vi "Rearrange image (20-02-2018).vi"(7 "Reference position":T2, 8 "error in (no error)":errorcluster, 9 "String ref array":refnum<vi>[](array[refnum]), 10 "Image refnum array":refnum<vi>[](array[refnum]), 11 "Image resize cluster":T3={"Image array"=[{"Size"={"Width"=500, "Height"=400}, "Position"={"Left"=0, "Top"=0}}, {"Size"={"Width"=500, "Height"=400}, "Position"={"Left"=0, "Top"=440}}, {"Size"={"Width"=500, "Height"=840}, "Position"={"Left"=505, "Top"=0}}], "String array"=[{"Size"={"Width"=503, "Height"=30}, "Position"={"Left"=0, "Top"=-30}}, {"Size"={"Width"=503, "Height"=30}, "Position"={"Left"=0, "Top"=410}}, {"Size"={"Width"=503, "Height"=30}, "Position"={"Left"=505, "Top"=-30}}]}) -> (0 "error out (no error)":errorcluster)   [LabVIEW 2015]
uses:
  Type Definitions/Controls and Indicators/String2.ctl
  <vilib>/Utility/miscctls.llb/LVPositionTypeDef.ctl
  <vilib>/Utility/miscctls.llb/LVBoundsTypeDef.ctl
  ZenGage v3.0 UI.lvclass
panel:
  out "Top Left 5":T4(plugin-control)
  out "Top Left 6":T5
  out "Top Left 3":T4(plugin-control)
  out "Top Left 4":T5
  out "Top Left 2":T4(plugin-control)
  out "Top Left":T5
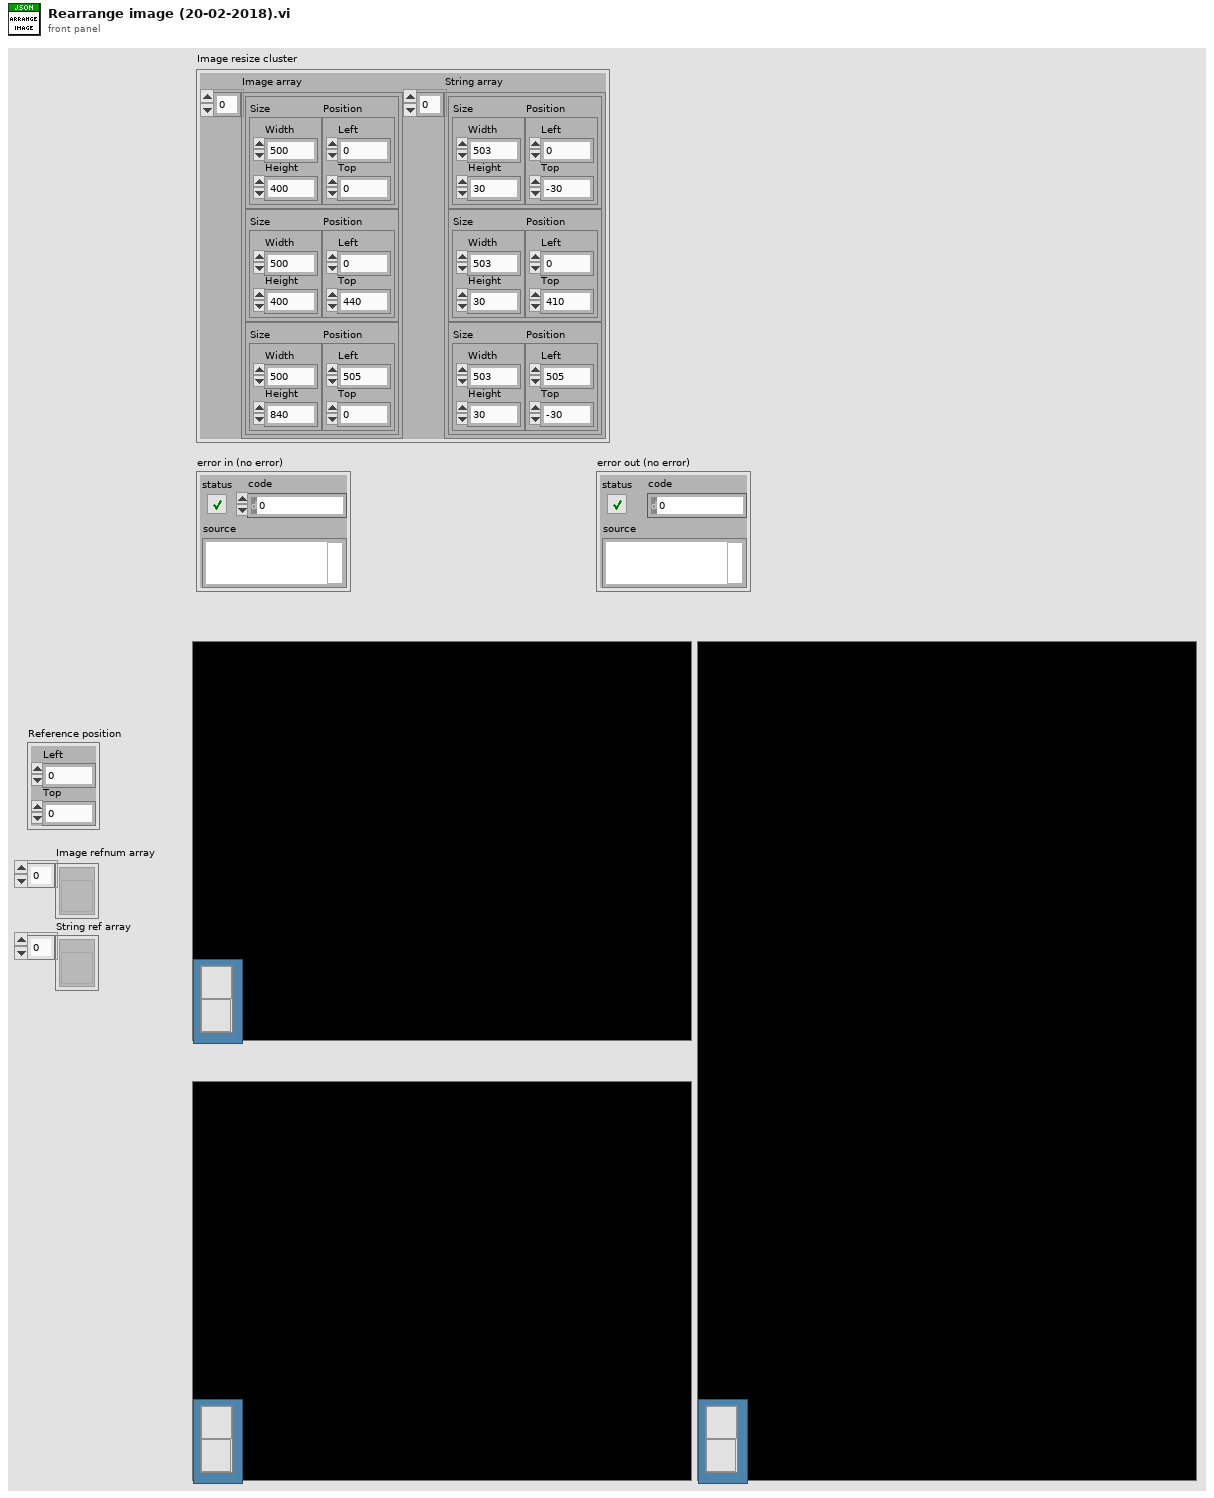
[diagram p1: front panel]
types:
  T1 = typedef "LVBoundsTypeDef.ctl" = cluster{"Width":u32, "Height":u32}
  T2 = typedef "LVPositionTypeDef.ctl" = cluster{"Left":i32, "Top":i32}
  T3 = cluster{"Image array":cluster{"Size":T1, "Position":T2}[], "String array":cluster{"Size":T1, "Position":T2}[]}
  T4 = typedef "IMAQ Image.ctl" = refnum<image>
  T5 = typedef "ZenGage v3.0 UI.lvclass/String2.ctl" = string
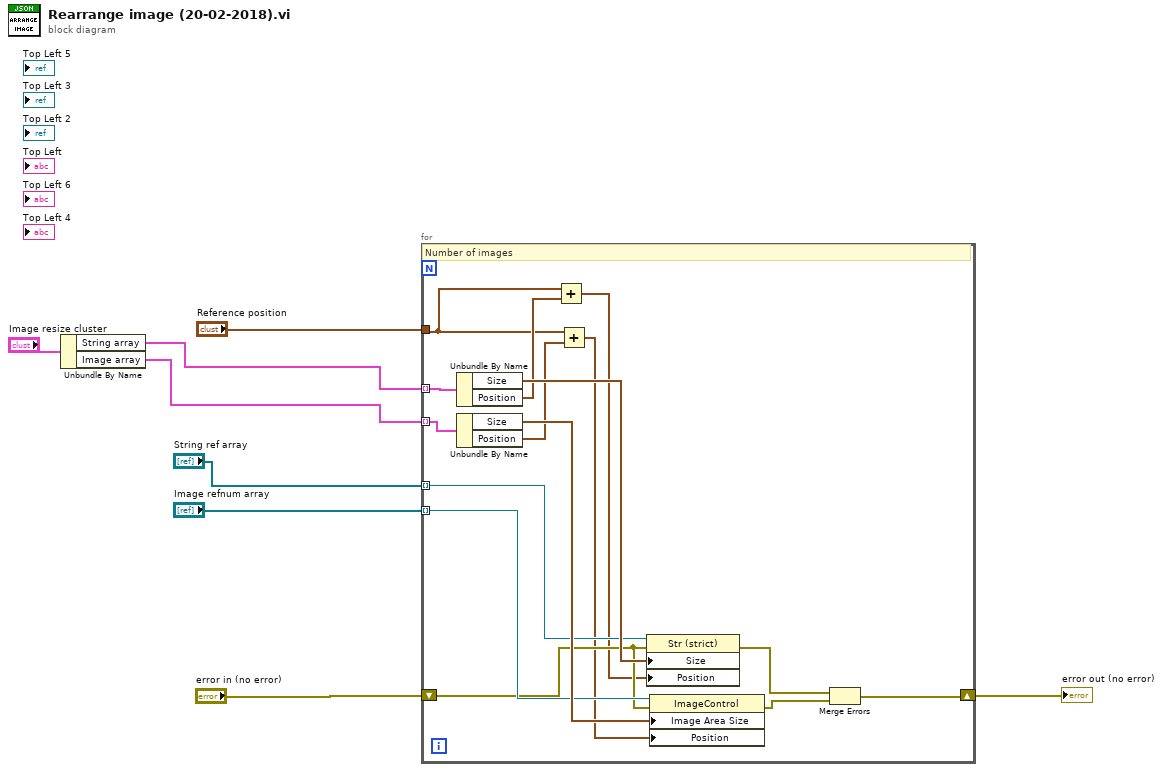
[diagram p0: block diagram]
diagram:
  n1 = Unbundle By Name("Image resize cluster") -> ("String array"=w4:cluster{"Size":T1, "Position":T2}[], "Image array"=w3:cluster{"Size":T1, "Position":T2}[])
  n2 = for {
    tunnel: "String ref array" -> [w19] mode=indexing
    tunnel: "Image refnum array" -> [w18] mode=indexing
    tunnel: w4 -> [w23] mode=indexing
    tunnel: w3 -> [w22] mode=indexing
    shift-right: [w14] -> w7
    shift-left: "error in (no error)" -> [w17]
    tunnel: "Reference position" -> [w12]
    # "Number of images"
    n3 = Unbundle By Name(w23) -> ("Size"=w21:T1, "Position"=w13:T2)
    n4 = Unbundle By Name(w22) -> ("Size"=w20:T1, "Position"=w11:T2)
    n5 = Add(x=w12, y=w13) -> (x+y=w10:T2)
    n6 = Add(x=w12, y=w11) -> (x+y=w9:T2)
    n7 = property class="Str (strict)"(reference=w19, error in=w17, "Size"=w21, "Position"=w10) -> (error out=w15:errorcluster)  [unwired: 1 out]
    n8 = property class="ImageControl"(reference=w18, error in=w17, "Image Area Size"=w20, "Position"=w9) -> (error out=w16:errorcluster)  [unwired: 1 out]
    n9 = Merge Errors(w15, w16) -> (w14:errorcluster)
  }
  "error out (no error)" <- w7
